vi "GenFunc_TU.vi"() -> ()   [LabVIEW 2025]
panel:
  in  "stop":bool
  out "size(s)":i32
  out "error out":errorcluster
  out "signal out":waveform(dbl)(graph)
  in  "error in (no error)":errorcluster
  in  "signal type":T1(ring)
  in  "noiseRMS":dbl=1.0 format="%.2p"
  in  "frequency":dbl=10.0 format="%0.2p"
  in  "amplitude":dbl=1.0 format="%0.2p"
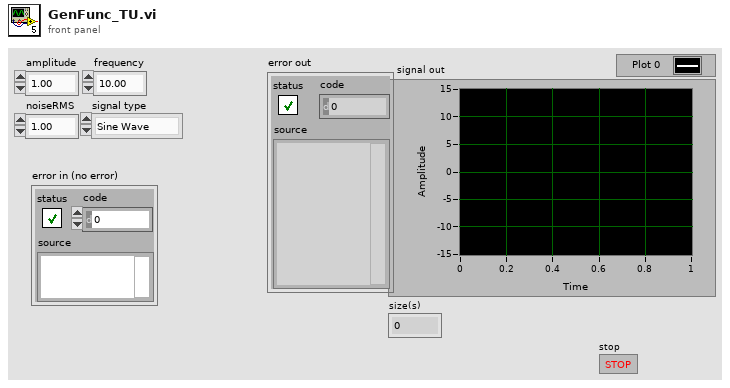
[diagram p1: front panel]
types:
  T1 = enum16{"Sine Wave", "Triangle Wave", "Square Wave", "Sawtooth Wave"}
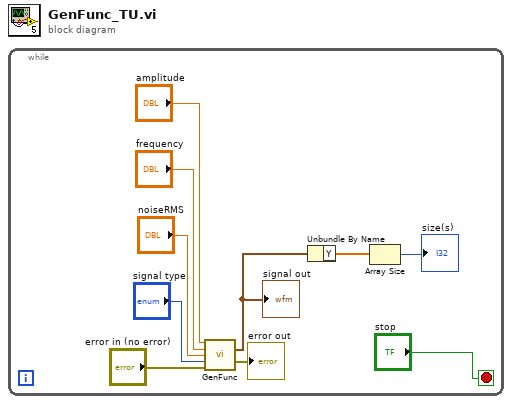
[diagram p0: block diagram]
diagram:
  n1 = while {
    stop <- "stop" stop-if-true
    n2 = call "GenFunc.vi"("amplitude"="amplitude", "frequency"="frequency", "noiseRMS"="noiseRMS", "signal type"="signal type", "error in (no error)"="error in (no error)") -> ("signal out"=w4:waveform(dbl), "error out"=→"error out":errorcluster)  [unwired: 9 in]
    "signal out" <- w4
    n3 = Unbundle By Name(w4) -> ("Y"=w3:dbl[])
    n4 = Array Size(array=w3) -> (size(s)=→"size(s)":i32)
  }
